vi "Finish.vi"   [LabVIEW 2013]
doc: "This VI is called just before exiting. It is expected to close I/O refnum, save collected data, etc."
uses:
  <vilib>/Rock Robotics/WPI/Joystick/WPI_JoystickGetSetRefNum.vi
  <vilib>/Rock Robotics/WPI/RobotDrive/WPI_RobotDriveGetSetRefNum.vi
types:
  T1 = typedef "WPI_JoystickDevRef.ctl" = cluster{"Device":T2}
  T2 = typedef "WPI_JoystickDeviceEnum.ctl" = enum16{"USB 1", "USB 2", "USB 3", "USB 4", "Kinect 1", "Kinect 2"}
  T3 = typedef "WPI_MotorControlDeviceRef.ctl" = cluster{"DeviceStatus":errorcluster, "Type":enum16{"PWM", "CAN"}, "PWM":cluster{"Digital Module":T4, "PWM Channel":T5, "DeadBand":T6}, "CAN":cluster{"Device Number":u8, "Control Mode":T7, "Semaphore":T8, "Max Vout":dbl}, "Invert":bool, "TransformRef":T9, "InvTransformRef":T9}
  T4 = typedef "FPGA_TypedefDigitalModule.ctl" = enum16{"Digital Module 1", "Digital Module 2"}
  T5 = typedef "FPGA_DIOPWMChannel.ctl" = enum8{"PWM 1", "PWM 2", "PWM 3", "PWM 4", "PWM 5", "PWM 6", "PWM 7", "PWM 8", "PWM 9", "PWM 10", "Invalid"}
  T6 = typedef "WPI_PWMDeadband.ctl" = cluster{"Name":string, "maxPositivePwm":i32, "minPositivePwm":i32, "centerPwm":i32, "maxNegativePwm":i32, "minNegativePwm":i32, "angularRange":u16}
  T7 = typedef "WPI_CANJaguar_ControlMode.ctl" = enum8{"Percent VBus", "Current", "Speed", "Position", "Voltage"}
  T8 = typedef "Semaphore RefNum" = refnum<k1>
  T9 = typedef "WPI_PWMTransform_ConPane.ctl" = refnum<vi>
  T10 = typedef "WPI_ServoDeviceRef.ctl" = cluster{"DeviceStatus":errorcluster, "Digital Module":T4, "PWM Channel":T5, "DeadBand":T6}
  T11 = typedef "WPI_RobotDriveDevRef.ctl" = cluster{"DevStatus":errorcluster, "Motors[]":T3[], "Square Inputs":bool, "Max Output":dbl, "Isochronous":bool}
  T12 = typedef "WPI_SolenoidDevRef.ctl" = cluster{"DevStatus":errorcluster, "Solenoid Module":T13, "Forward Solenoid Channel":T14, "Reverse Solenoid Channel":T14}
  T13 = typedef "FPGA_TypedefSolenoidModule.ctl" = enum16{"Solenoid Module 1", "Solenoid Module 2"}
  T14 = typedef "WPI_SolenoidChannel.ctl" = enum8{"Solenoid 1", "Solenoid 2", "Solenoid 3", "Solenoid 4", "Solenoid 5", "Solenoid 6", "Solenoid 7", "Solenoid 8", "Invalid"}
  T15 = typedef "WPI_DigitalInputDevRef.ctl" = cluster{"DevStatus":errorcluster, "DIO Channel":T16, "Digital Module":T4}
  T16 = typedef "FPGA_DIOChannel.ctl" = enum8{"DIO 1", "DIO 2", "DIO 3", "DIO 4", "DIO 5", "DIO 6", "DIO 7", "DIO 8", "DIO 9", "DIO 10", "DIO 11", "DIO 12", "DIO 13", "DIO 14", "Invalid"}
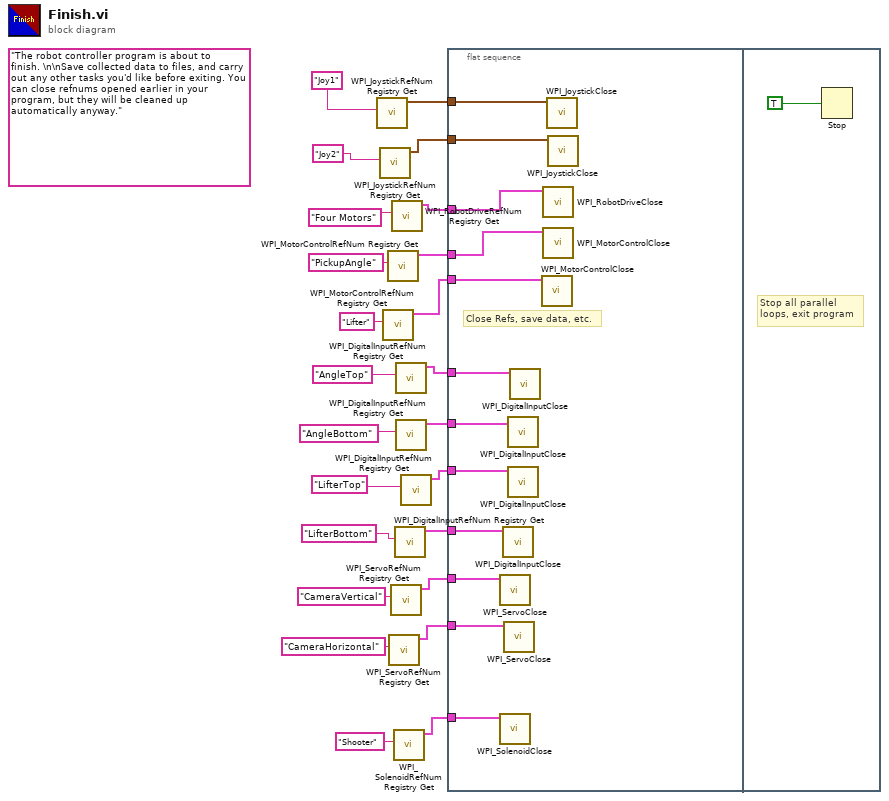
[diagram p0: block diagram]
diagram:
  (unwired) "The robot controller program is about to finish. \n\nSave collected data to files, and carry out any other tasks you'd like before exiting. You can close refnums opened earlier in your program, but they will be cleaned up automatically anyway."
  n1 = call <vilib>:"WPI_JoystickRefNum Registry Get.vi"("refnum name"="Joy1") -> ("JoystickDevRef"=w21:T1)  [unwired: 1 in, 9 out]
  n2 = call <vilib>:"WPI_JoystickRefNum Registry Get.vi"("refnum name"="Joy2") -> ("JoystickDevRef"=w19:T1)  [unwired: 1 in, 9 out]
  n3 = call <vilib>:"WPI_MotorControlRefNum Registry Get.vi"("refnum name"="Lifter") -> ("MotorControlDevRef"=w15:T3)  [unwired: 9 in, 1 out]
  n4 = call <vilib>:"WPI_MotorControlRefNum Registry Get.vi"("refnum name"="PickupAngle") -> ("MotorControlDevRef"=w16:T3)  [unwired: 9 in, 1 out]
  n5 = call <vilib>:"WPI_ServoRefNum Registry Get.vi"("refnum name"="CameraHorizontal") -> ("ServoDeviceRef"=w3:T10)  [unwired: 9 in, 1 out]
  n6 = call <vilib>:"WPI_ServoRefNum Registry Get.vi"("refnum name"="CameraVertical") -> ("ServoDeviceRef"=w4:T10)  [unwired: 9 in, 1 out]
  n7 = call <vilib>:"WPI_RobotDriveRefNum Registry Get.vi"("refnum name"="Four Motors") -> ("RobotDriveDevRef"=w22:T11)  [unwired: 1 in, 9 out]
  n8 = call <vilib>:"WPI_SolenoidRefNum Registry Get.vi"("refnum name"="Shooter") -> ("SolenoidDevRef"=w2:T12)  [unwired: 9 in, 1 out]
  n9 = call <vilib>:"WPI_DigitalInputRefNum Registry Get.vi"("refnum name"="LifterBottom") -> ("DigitalInputDevRef"=w7:T15)  [unwired: 9 in, 1 out]
  n10 = call <vilib>:"WPI_DigitalInputRefNum Registry Get.vi"("refnum name"="AngleTop") -> ("DigitalInputDevRef"=w10:T15)  [unwired: 9 in, 1 out]
  n11 = call <vilib>:"WPI_DigitalInputRefNum Registry Get.vi"("refnum name"="AngleBottom") -> ("DigitalInputDevRef"=w9:T15)  [unwired: 9 in, 1 out]
  n12 = call <vilib>:"WPI_DigitalInputRefNum Registry Get.vi"("refnum name"="LifterTop") -> ("DigitalInputDevRef"=w8:T15)  [unwired: 9 in, 1 out]
  n13 = flat-sequence {
    tunnel: w22 -> [w36]
    tunnel: w21 -> [w35]
    tunnel: w19 -> [w34]
    tunnel: w16 -> [w33]
    tunnel: w15 -> [w32]
    tunnel: w10 -> [w31]
    tunnel: w9 -> [w30]
    tunnel: w8 -> [w29]
    tunnel: w7 -> [w28]
    tunnel: w4 -> [w27]
    tunnel: w3 -> [w26]
    tunnel: w2 -> [w25]
    frame #0 {
      # "Close Refs, save data, etc."
      n14 = call <vilib>:"WPI_ServoClose.vi"("MotorControlDevRef"=w27) -> ()  [unwired: 10 in, 1 out]
      n15 = call <vilib>:"WPI_SolenoidClose.vi"("SolenoidDevRef"=w25) -> ()  [unwired: 10 in, 1 out]
      n16 = call <vilib>:"WPI_DigitalInputClose.vi"("DigitalInputDevRef"=w28) -> ()  [unwired: 10 in, 1 out]
      n17 = call <vilib>:"WPI_ServoClose.vi"("MotorControlDevRef"=w26) -> ()  [unwired: 10 in, 1 out]
      n18 = call <vilib>:"WPI_DigitalInputClose.vi"("DigitalInputDevRef"=w30) -> ()  [unwired: 10 in, 1 out]
      n19 = call <vilib>:"WPI_DigitalInputClose.vi"("DigitalInputDevRef"=w29) -> ()  [unwired: 10 in, 1 out]
      n20 = call <vilib>:"WPI_DigitalInputClose.vi"("DigitalInputDevRef"=w31) -> ()  [unwired: 10 in, 1 out]
      n21 = call <vilib>:"WPI_MotorControlClose.vi"("MotorControlDevRef"=w32) -> ()  [unwired: 10 in, 1 out]
      n22 = call <vilib>:"WPI_RobotDriveClose.vi"("RobotDriveDevRef"=w36) -> ()  [unwired: 1 in, 10 out]
      n23 = call <vilib>:"WPI_MotorControlClose.vi"("MotorControlDevRef"=w33) -> ()  [unwired: 10 in, 1 out]
      n24 = call <vilib>:"WPI_JoystickClose.vi"("JoystickDevRef"=w35) -> ()  [unwired: 11 out]
      n25 = call <vilib>:"WPI_JoystickClose.vi"("JoystickDevRef"=w34) -> ()  [unwired: 11 out]
    }
    frame #1 {
      # "Stop all parallel\nloops, exit program"
      n26 = Stop(stop? (T)=TRUE ("Quit")) -> ()
    }
  }
